vi "客户端侦听列表.vi"() -> ()   [LabVIEW 2016, in "wxpusher.lvlib"]
uses:
  wxpusher.lvlib
  <vilib>/Utility/miscctls.llb/LVPointTypeDef.ctl
  <vilib>/httpClient/LabVIEWHTTPClient.lvlib
panel:
  out "数据输出":string
  in  "开机启动":bool
  out "remote port":u16
  out "remote address":string
  out "data out":string
  out "数组":refnum<k5>[](array[refnum])
  out "回调信息":T1
  out "侦听列表":T2(array[cluster])
  in  "客户端列表":i32(listbox)
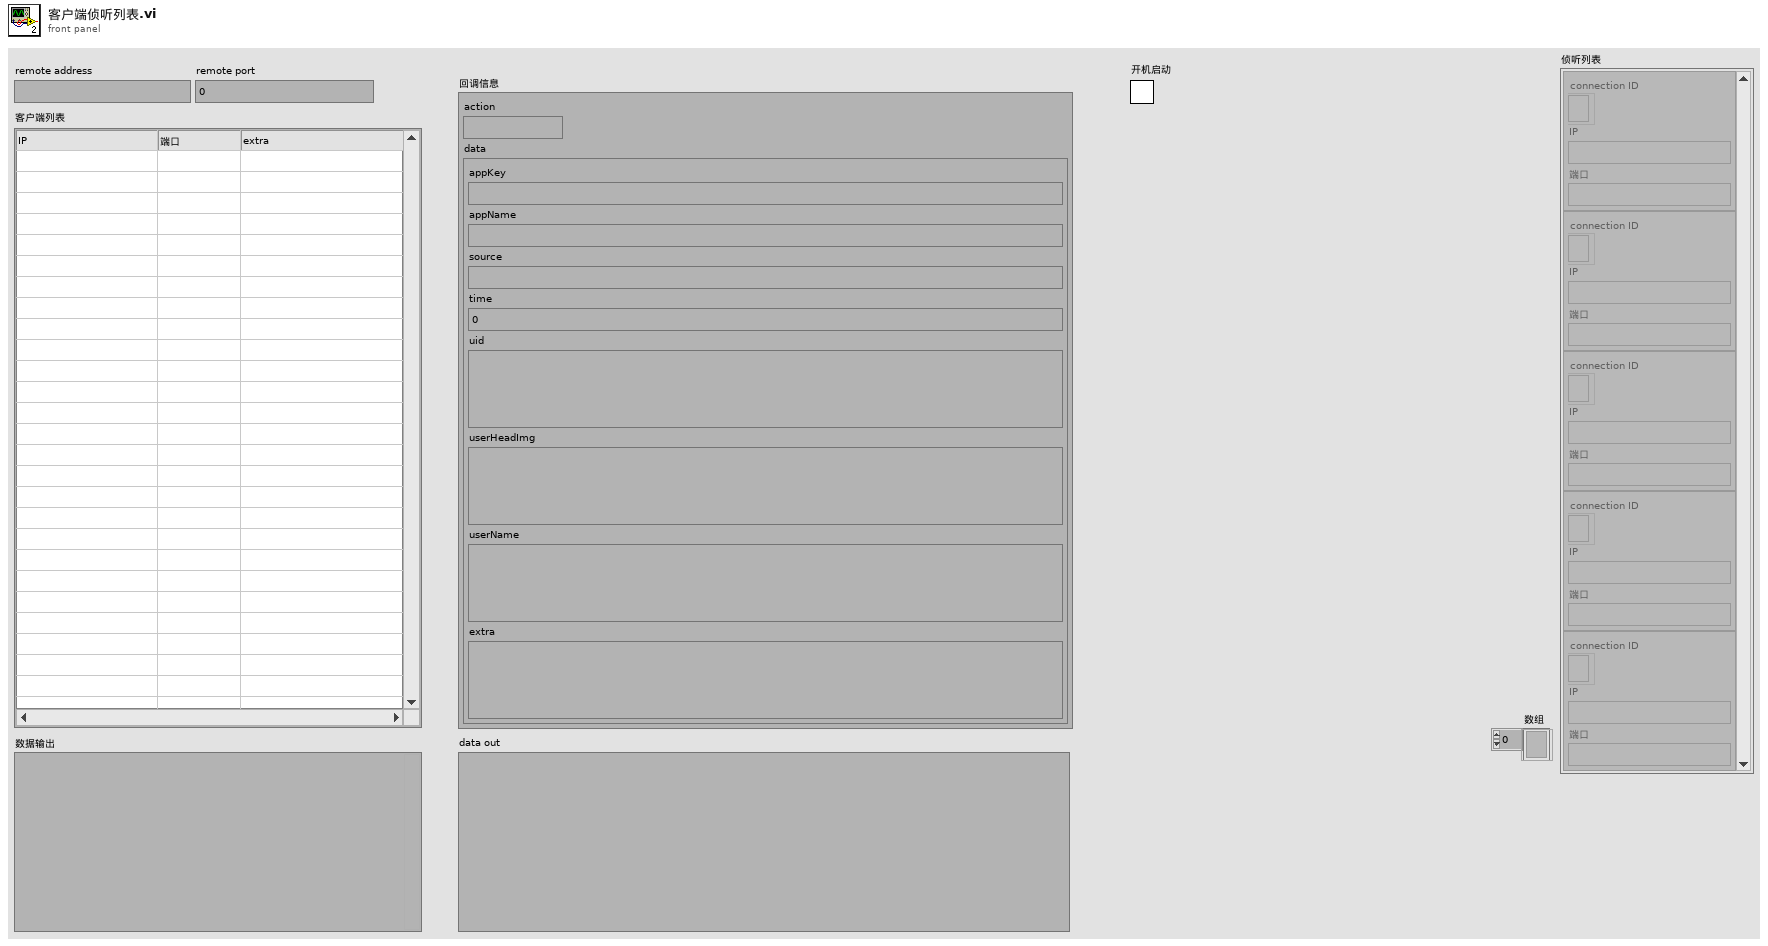
[diagram p1: front panel]
types:
  T1 = cluster{"action":string, "data":cluster{"appKey":string, "appName":string, "source":string, "time":u64, "uid":string, "userHeadImg":string, "userName":string, "extra":string}}
  T2 = cluster{"connection ID":refnum<k5>, "IP":string, "端口":string}[]
  T3 = typedef "LVPointTypeDef.ctl" = cluster{"Horizontal":i16, "Vertical":i16}
  T4 = cluster{"数据输出":string, "data":cluster{"action":string, "data":cluster{"appKey":string, "appName":string, "source":string, "time":u64, "uid":string, "userHeadImg":string, "userName":string, "extra":string}}}
  T5 = cluster{"connection ID":refnum<k5>, "IP":string, "端口":string}
  T6 = cluster{"cmd":string, "data":cluster{"png":u8[]}}
  T7 = enum16{"Standard", "Buffered", "CRLF", "Immediate"}
  T8 = typedef "LabVIEWHTTPClient.lvlib/ClientHandle.ctl" = refnum<k1>
  T9 = cluster{"data out":string, "类型和默认值":cluster{"action":string, "data":cluster{"appKey":string, "appName":string, "source":string, "time":u64, "uid":string, "userHeadImg":string, "userName":string, "extra":string}}}
  T10 = cluster{"cmd":string, "data":cluster{"action":string, "data":cluster{"appKey":string, "appName":string, "source":string, "time":u64, "uid":string, "userHeadImg":string, "userName":string, "extra":string}}}
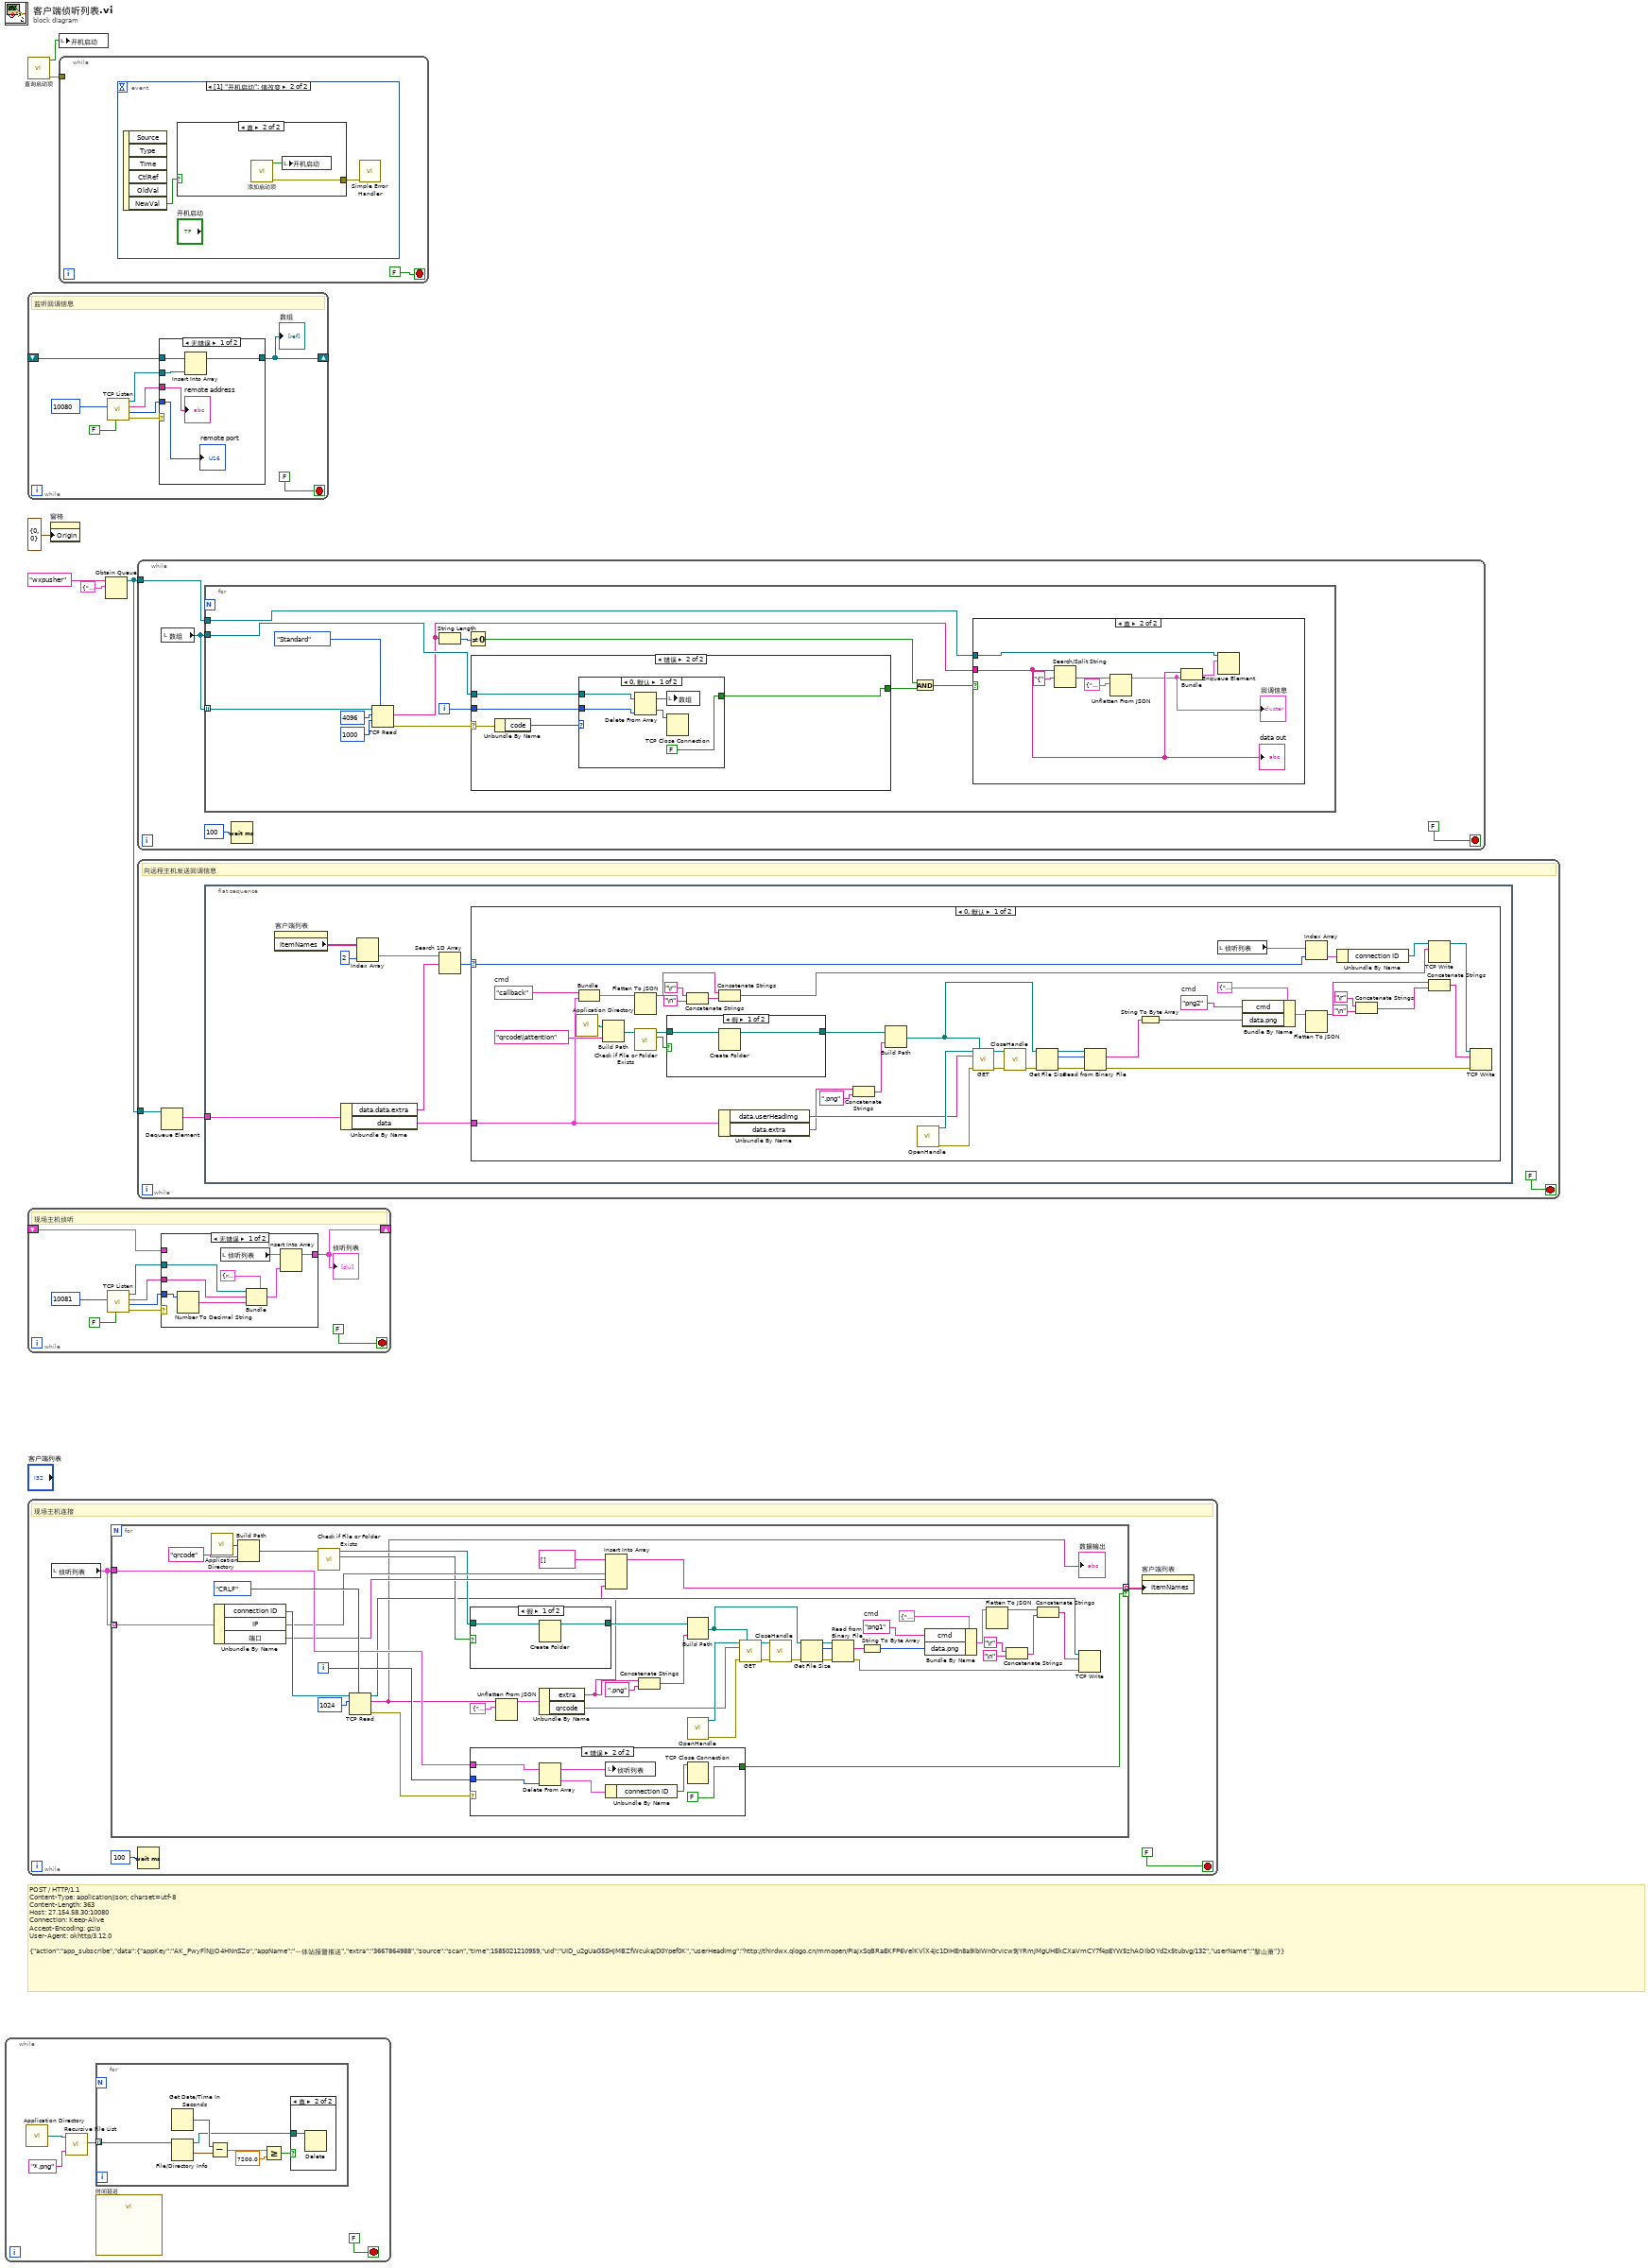
[diagram p0: block diagram]
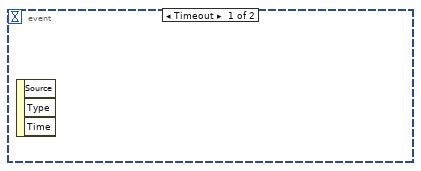
[diagram p3: hidden frame]
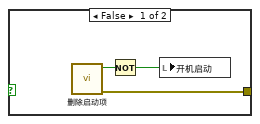
[diagram p4: hidden frame]
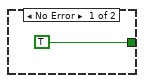
[diagram p6: hidden frame]
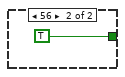
[diagram p7: hidden frame]
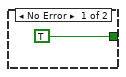
[diagram p12: hidden frame]
diagram:
  # "POST / HTTP/1.1\nContent-Type: application/json; charset=utf-8\nContent-Length: 363\nHost: 27.154.58.30:10080\nConnection: Keep-Alive\nAccept-Encoding: gzip\nUser-Agent: okhttp/3.12.0\n\n{\"action\":\"app_subscribe\",\"data\":{\"appKey\":\"AK_PwyFlNJjO4HNnSZo\",\"appName\":\"一体站报警推送\",\"extra\":\"3667864988\",\"source\":\"scan\",\"time\":1585021210959,\"uid\":\"UID_u2gUaG5SHjMBZfWcukaJD0Ypef0K\",\"userHeadImg\":\"http://thirdwx.qlogo.cn/mmopen/PiajxSqBRaEKFP6VelKVlX4Jc1DIHEn8a9ibIWn0rvicw9jYRmJMgUHEkCXaVmCY7f4pEYW5zhAOIbOYd2x5tubvg/132\",\"userName\":\"黎山萧\"}}"
  n1 = while {
    stop <- FALSE stop-if-true
    n2 = call <vilib>:"Application Directory.vi"() -> ("Application Directory"=w9:path)
    n3 = call <vilib>:"Recursive File List.vi"("pattern"="*.png", "Folder Path"=w9) -> ("All Files in Dir"=w7:path[])  [unwired: 5 in, 4 out]
    n4 = for {
      tunnel: w7 -> [w17] mode=indexing
      n5 = Get Date/Time In Seconds() -> (seconds since 1Jan1904=w15:timestamp)
      n6 = File/Directory Info(path=w17) -> (path out=w11:path, last mod=w16:timestamp)  [unwired: 1 in, 5 out]
      n7 = Subtract(x=w15, y=w16) -> (x-y=w14:dbl)
      n8 = Greater Or Equal?(x=w14, y=7200.0) -> (x >= y?=w12:bool)
      n9 = case shown="真" w12 {
        tunnel: w11 -> [_ w18]
        frame False {
        }
        frame True {
          n10 = Delete(path (use dialog)=w18) -> ()  [unwired: 4 in, 3 out]
        }
      }
    }
    n11 = call "时间延迟"() -> ()  [unwired: 11 in, 1 out]
  }
  n12 = call "查询启动项.vi"() -> ("error out"=w3:errorcluster, "包含启动项"=w2:bool)  [unwired: 9 in, 1 out]
  n13 = while {
    shift-right: [w22] -> _
    shift-left: _ -> [w21]
    stop <- FALSE stop-if-true
    # "监听回调信息"
    n14 = call <vilib>:"TCP Listen.vi"("resolve remote address (T)"=FALSE, "port"=u16 10080) -> ("error out"=w25:errorcluster, "remote port"=w19:u16, "remote address"=w24:string, "connection ID"=w23:refnum<k5>)  [unwired: 5 in, 1 out]
    n15 = case shown="无错误" w25 {
      tunnel: w23 -> [w32 _]
      tunnel: w24 -> [w29 _]
      tunnel: [w31 w33] -> w22
      tunnel: w21 -> [w30 w33]
      tunnel: w19 -> [w28 _]
      frame No Error {
        n16 = Insert Into Array(array=w30, new element=w32) -> (w31:refnum<k5>[])  [unwired: 1 in]
        "remote address" <- w29
        "remote port" <- w28
      }
      frame Error {
      }
    }
    "数组" <- w22
  }
  n17 = while {
    shift-right: [w36] -> _
    shift-left: _ -> [w35]
    stop <- FALSE stop-if-true
    # "现场主机侦听"
    n18 = call <vilib>:"TCP Listen.vi"("resolve remote address (T)"=FALSE, "port"=u16 10081) -> ("error out"=w40:errorcluster, "remote port"=w37:u16, "remote address"=w38:string, "connection ID"=w39:refnum<k5>)  [unwired: 5 in, 1 out]
    n19 = case shown="无错误" w40 {
      tunnel: w39 -> [w50 _]
      tunnel: w38 -> [w44 _]
      tunnel: w37 -> [w45 _]
      tunnel: [w48 w51] -> w36
      tunnel: w35 -> [_ w51]
      frame No Error {
        n20 = Number To Decimal String(number=w45) -> (decimal integer string=w47:string)  [unwired: 1 in]
        n21 = local read "侦听列表"() -> (w43:T2)
        n22 = Bundle(cluster=T5 {"connection ID"=refnum, "IP"="", "端口"=""} ("簇"), "connection ID"=w50, "IP"=w44, "端口"=w47) -> (w49:T5)
        n23 = Insert Into Array(array=w43, new element=w49) -> (w48:T2)  [unwired: 1 in]
      }
      frame Error {
      }
    }
    "侦听列表" <- w36
  }
  n24 = while {
    stop <- FALSE stop-if-true
    # "现场主机连接"
    n25 = local read "侦听列表"() -> (w53:T2)
    n26 = for {
      tunnel: w53 -> [w101] mode=indexing
      tunnel: [w91] -> w52 mode=indexing if=w95
      tunnel: w53 -> [w97]
      i -> [w96]
      w58 = "png1"  # cmd
      n27 = call <vilib>:"Application Directory.vi"() -> ("Application Directory"=w71:path)
      n28 = Unbundle By Name(w101) -> ("connection ID"=w100:refnum<k5>, "IP"=w94:string, "端口"=w93:string)
      n29 = Build Path(base path=w71, name or relative path="qrcode" ("名称或相对路径")) -> (appended path=w84:path)
      n30 = call <vilib>:"Check if File or Folder Exists.vi"("path"=w84) -> ("file or folder exists?"=w82:bool, "dup path"=w83:path)  [unwired: 8 in, 1 out]
      n31 = TCP Read(connection ID=w100, bytes to read=1024 ("读取的字节"), 7:T7."CRLF" ("模式（标准）")) -> (connection ID out=w73:refnum<k5>, data out=w67:string, error out=w90:errorcluster)  [unwired: 2 in]
      "数据输出" <- w67
      n32 = case shown="假" w82 {
        tunnel: [w103 w104] -> w85
        tunnel: w83 -> [w102 w104]
        frame False {
          n33 = Create Folder(path (use dialog)=w102) -> (created path=w103:path)  [unwired: 2 in, 2 out]
        }
        frame True {
        }
      }
      n34 = case shown="错误" w90 {
        tunnel: w97 -> [_ w111]
        tunnel: w96 -> [_ w110]
        tunnel: [TRUE FALSE] -> w95
        frame No Error {
        }
        frame Error {
          n35 = Delete From Array(array=w111, index=w110) -> (deleted portion=w107:T5, array with subset deleted=w108:T2)  [unwired: 1 in]
          n36 = local write "侦听列表"(w108) -> ()
          n37 = Unbundle By Name(w107) -> ("connection ID"=w106:refnum<k5>)
          n38 = TCP Close Connection(connection ID=w106) -> ()  [unwired: 2 in, 2 out]
        }
      }
      n39 = Unflatten From JSON(JSON string=w67, type and defaults=cluster{"extra":string, "qrcode":string} {"extra"="", "qrcode"=""}) -> (value=w65:cluster{"extra":string, "qrcode":string})  [unwired: 5 in, 1 out]
      n40 = Unbundle By Name(w65) -> ("extra"=w63:string, "qrcode"=w64:string)
      n41 = Insert Into Array(array=string[] [] ("数组"), new element #1=w94, new element #2=w93, new element #3=w63) -> (w91:string[])  [unwired: 1 in]
      n42 = Concatenate Strings(w63, ".png" ("字符串")) -> (w79:string)
      n43 = Build Path(base path=w85, name or relative path=w79) -> (appended path=w78:path)
      n44 = call <vilib>:"OpenHandle.vi"() -> ("client handle out"=w89:T8, "error out"=w88:errorcluster)  [unwired: 14 in]
      n45 = call <vilib>:"GET.vi"("client handle"=w89, "output file"=w78, "url"=w64, "error in (no error)"=w88) -> ("client handle out"=w87:T8, "error out"=w86:errorcluster)  [unwired: 8 in, 2 out]
      n46 = call <vilib>:"CloseHandle.vi"("client handle"=w87, "error in (no error)"=w86) -> ("error out"=w76:errorcluster)  [unwired: 13 in]
      n47 = Get File Size(file=w78, error in=w76) -> (refnum out=w77:refnum<file>, size (in bytes)=w74:i64, 0:w75:errorcluster)
      n48 = Read from Binary File(8:w75, 10:w74, 11:w77) -> (0:w72:errorcluster, 2:w57:string)  [unwired: 3 in, 2 out]
      n49 = String To Byte Array(string=w57) -> (unsigned byte array=w56:u8[])
      n50 = Bundle By Name(cluster=T6 {"cmd"="", "data"={"png"=[]}}, "cmd"=w58, "data.png"=w56) -> (w69:T6)
      n51 = Flatten To JSON(anything=w69) -> (JSON string=w68:string)  [unwired: 2 in, 1 out]
      n52 = Concatenate Strings("\r", "\n") -> (w59:string)
      n53 = Concatenate Strings(w68, w59) -> (w62:string)
      n54 = TCP Write(connection ID=w73, data in=w62, error in (no error)=w72) -> ()  [unwired: 1 in, 3 out]
    }
    n55 = Wait (ms)(milliseconds to wait=u32 100 ("等待时间（毫秒）")) -> ()  [unwired: 1 out]
    n56 = property on="客户端列表" class="MCListbox (严格)"("ItemNames"=w52) -> ()  [unwired: 2 in, 2 out]
  }
  n57 = property on="窗格" class="Pane"("Origin"=T3 {"Horizontal"=0, "Vertical"=0} ("原点")) -> ()  [unwired: 2 in, 2 out]
  n58 = local write "开机启动"(w2) -> ()
  n59 = while {
    tunnel: w3 -> [_]
    stop <- FALSE stop-if-true
    n60 = event shown="[1] \"开机启动\": 值改变" {
      selector: _ -> [_ _]
      dyn-events: _ -> [_ _]
      timeout: _ -> [_ _]
      event Timeout {
        n61 = event-data() -> ()  [unwired: 1 in, 3 out]
      }
      event "开机启动": Value Change {
        n62 = event-data() -> ("NewVal"=w114:bool)  [unwired: 1 in, 5 out]
        n63 = case shown="真" w114 {
          tunnel: [w115 w118] -> w113
          frame False {
            n64 = call "删除启动项.vi"() -> ("error out"=w115:errorcluster, "删除标记"=w117:bool)  [unwired: 10 in]
            n65 = Not(x=w117) -> (.not. x?=w116:bool)
            n66 = local write "开机启动"(w116) -> ()
          }
          frame True {
            n67 = call "添加启动项.vi"() -> ("error out"=w118:errorcluster, "添加成功标记"=w119:bool)  [unwired: 10 in]
            n68 = local write "开机启动"(w119) -> ()
          }
        }
        n69 = call <vilib>:"Simple Error Handler.vi"("error in (no error)"=w113) -> ()  [unwired: 4 in, 5 out]
      }
    }
  }
  n70 = Obtain Queue(name (unnamed)="wxpusher" ("名称（未命名）"), element data type=T4 {"数据输出"="", "data"={"action"="", "data"={"appKey"="", "appName"="", "source"="", "time"=0, "uid"="", "userHeadImg"="", "userName"="", "extra"=""}}}) -> (queue out=w4:refnum<queue>)  [unwired: 3 in, 2 out]
  n71 = while {
    tunnel: w4 -> [w122]
    stop <- FALSE stop-if-true
    n72 = local read "数组"() -> (w120:refnum<k5>[])
    n73 = for {
      tunnel: w122 -> [w136]
      tunnel: w120 -> [w132] mode=indexing
      tunnel: w120 -> [w129]
      i -> [w131]
      n74 = TCP Read(connection ID=w132, bytes to read=4096 ("读取的字节"), 7:T7."Standard" ("模式（标准）"), 9:1000 ("超时毫秒(25000)")) -> (data out=w127:string, error out=w130:errorcluster)  [unwired: 1 in, 1 out]
      n75 = String Length(string=w127) -> (length=w126:i32)
      n76 = Not Equal To 0?(x=w126) -> (x != 0?=w124:bool)
      n77 = case shown="错误" w130 {
        selector: w130 -> [_ w149]
        tunnel: w129 -> [_ w147]
        tunnel: w131 -> [_ w146]
        tunnel: [TRUE w145] -> w128
        frame No Error {
        }
        frame Error {
          n78 = Unbundle By Name(w149) -> ("code"=w148:i32)
          n79 = case shown="0, 默认" w148 {
            tunnel: w147 -> [w154 _]
            tunnel: w146 -> [w153 _]
            tunnel: [FALSE TRUE] -> w145
            frame 0, Default {
              n80 = Delete From Array(array=w154, index=w153) -> (deleted portion=w150:refnum<k5>, array with subset deleted=w152:refnum<k5>[])  [unwired: 1 in]
              n81 = local write "数组"(w152) -> ()
              n82 = TCP Close Connection(connection ID=w150) -> ()  [unwired: 2 in, 2 out]
            }
            frame 56 {
            }
          }
        }
      }
      n83 = And(x=w124, y=w128) -> (x .and. y?=w125:bool)
      n84 = case shown="真" w125 {
        tunnel: w136 -> [_ w143]
        tunnel: w127 -> [_ w142]
        frame False {
        }
        frame True {
          n85 = Search/Split String(string=w142, search string/char (-)="{" ("搜索字符串/字符(-)")) -> (match + rest of string=w139:string)  [unwired: 1 in, 2 out]
          n86 = Unflatten From JSON(JSON string=w139, type and defaults=T1 {"action"="", "data"={"appKey"="", "appName"="", "source"="", "time"=0, "uid"="", "userHeadImg"="", "userName"="", "extra"=""}} ("类型和默认值")) -> (value=w138:T1)  [unwired: 5 in, 1 out]
          "回调信息" <- w138
          n87 = Bundle("data out"=w142, "类型和默认值"=w138) -> (w137:T9)  [unwired: 1 in]
          n88 = Enqueue Element(queue=w143, element=w137) -> ()  [unwired: 2 in, 3 out]
          "data out" <- w142
        }
      }
    }
    n89 = Wait (ms)(milliseconds to wait=u32 100 ("等待时间（毫秒）")) -> ()  [unwired: 1 out]
  }
  n90 = while {
    tunnel: w4 -> [w158]
    stop <- FALSE stop-if-true
    # "向远程主机发送回调信息"
    n91 = Dequeue Element(queue=w158) -> (element=w156:T4)  [unwired: 2 in, 3 out]
    n92 = flat-sequence {
      tunnel: w156 -> [w165]
      frame #0 {
        n93 = property on="客户端列表" class="MCListbox (严格)"() -> ("ItemNames"=w164:string[][])  [unwired: 2 in, 2 out]
        n94 = Unbundle By Name(w165) -> ("data.data.extra"=w161:string, "data"=w159:T1)
        n95 = Index Array(array=w164, index (col)=2 ("禁用的索引 (列)")) -> (element=w162:string[])  [unwired: 1 in]
        n96 = Search 1D Array(1D array=w162, element=w161) -> (index of element=w160:i32)  [unwired: 1 in]
        n97 = case shown="0, 默认" w160 {
          selector: w160 -> [w207 _]
          tunnel: w159 -> [w199 _]
          frame 0, Default {
            w171 = "png2"  # cmd
            w198 = "callback"  # cmd
            n98 = call <vilib>:"Application Directory.vi"() -> ("Application Directory"=w179:path)
            n99 = Bundle("cmd"=w198, "data"=w199) -> (w197:T10)  [unwired: 1 in]
            n100 = Build Path(base path=w179, name or relative path="qrcode\\attention" ("名称或相对路径")) -> (appended path=w191:path)
            n101 = Flatten To JSON(anything=w197) -> (JSON string=w204:string)  [unwired: 2 in, 1 out]
            n102 = call <vilib>:"Check if File or Folder Exists.vi"("path"=w191) -> ("file or folder exists?"=w189:bool, "dup path"=w190:path)  [unwired: 8 in, 1 out]
            n103 = case shown="假" w189 {
              tunnel: [w210 w211] -> w192
              tunnel: w190 -> [w209 w211]
              frame False {
                n104 = Create Folder(path (use dialog)=w209) -> (created path=w210:path)  [unwired: 2 in, 2 out]
              }
              frame True {
              }
            }
            n105 = Concatenate Strings("\r", "\n") -> (w200:string)
            n106 = Concatenate Strings(w204, w200) -> (w203:string)
            n107 = Unbundle By Name(w199) -> ("data.userHeadImg"=w168:string, "data.extra"=w167:string)
            n108 = Concatenate Strings(w167, ".png" ("字符串")) -> (w186:string)
            n109 = Build Path(base path=w192, name or relative path=w186) -> (appended path=w185:path)
            n110 = call <vilib>:"OpenHandle.vi"() -> ("client handle out"=w196:T8, "error out"=w195:errorcluster)  [unwired: 14 in]
            n111 = call <vilib>:"GET.vi"("client handle"=w196, "output file"=w185, "url"=w168, "error in (no error)"=w195) -> ("client handle out"=w194:T8, "error out"=w193:errorcluster)  [unwired: 8 in, 2 out]
            n112 = call <vilib>:"CloseHandle.vi"("client handle"=w194, "error in (no error)"=w193) -> ("error out"=w183:errorcluster)  [unwired: 13 in]
            n113 = Get File Size(file=w185, error in=w183) -> (refnum out=w184:refnum<file>, size (in bytes)=w181:i64, 0:w182:errorcluster)
            n114 = Read from Binary File(8:w182, 10:w181, 11:w184) -> (0:w180:errorcluster, 2:w170:string)  [unwired: 3 in, 2 out]
            n115 = String To Byte Array(string=w170) -> (unsigned byte array=w169:u8[])
            n116 = local read "侦听列表"() -> (w208:T2)
            n117 = Bundle By Name(cluster=T6 {"cmd"="", "data"={"png"=[]}}, "cmd"=w171, "data.png"=w169) -> (w177:T6)
            n118 = Index Array(array=w208, index=w207) -> (element=w206:T5)
            n119 = Flatten To JSON(anything=w177) -> (JSON string=w176:string)  [unwired: 2 in, 1 out]
            n120 = Unbundle By Name(w206) -> ("connection ID"=w205:refnum<k5>)
            n121 = Concatenate Strings("\r", "\n") -> (w172:string)
            n122 = TCP Write(connection ID=w205, data in=w203) -> (connection ID out=w166:refnum<k5>)  [unwired: 2 in, 2 out]
            n123 = Concatenate Strings(w176, w172) -> (w175:string)
            n124 = TCP Write(connection ID=w166, data in=w175, error in (no error)=w180) -> ()  [unwired: 1 in, 3 out]
          }
          frame -1 {
          }
        }
      }
    }
  }
